vi "PH_Beckhoff_PP_PU.handle RRs.vi"(0 "i ref in":refnum<vi>, 4 "Values":T2, 5 "error in":errorcluster, 7 "Values changed at":T1) -> (14 "i ref out":refnum<vi>, 19 "error out":errorcluster)   [LabVIEW 2014, in "PH_Beckhoff_PP_PU.lvlib"]
doc: "This VI handles the incoming information about Ross Relais: The status is calculated and, if it changed, set to own attributes and published via DIM. All information is indicated at the GUI."
uses:
  PH_Beckhoff_PP_PU.lvlib
  PH_Beckhoff/PH_Beckhoff.Values.ctl
  PH_Beckhoff/PH_Beckhoff.Sonderklemmen Inputs.ctl
  PH_Beckhoff/PH_Beckhoff.Analog Inputs.ctl
  PH_Beckhoff/PH_Beckhoff.Scaling Type.ctl
  PH_Beckhoff/PH_Beckhoff.Analog Outputs.ctl
  PH_Beckhoff/PH_Beckhoff.Digital Inputs.ctl
  PH_Beckhoff/PH_Beckhoff.Digital Outputs.ctl
  PH_Basics/PH_StatusHandler/PH_StatusHandler.lvlib
  PH_Basics/PH_Common/PH_Common.lvlib
  PH_Beckhoff/PH_Beckhoff.lvlib
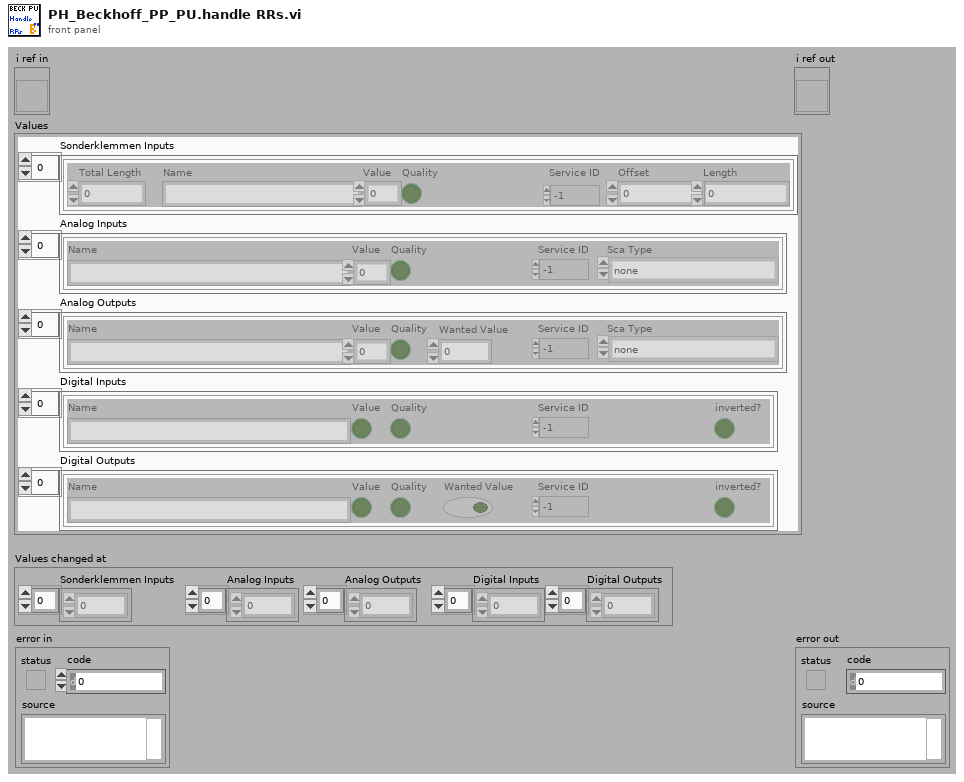
[diagram p1: front panel]
types:
  T1 = cluster{"Sonderklemmen Inputs":i32[], "Analog Inputs":i32[], "Analog Outputs":i32[], "Digital Inputs":i32[], "Digital Outputs":i32[]}
  T2 = typedef "PH_Beckhoff.lvlib/PH_Beckhoff.Values.ctl" = cluster{"Sonderklemmen Inputs":T3, "Analog Inputs":T4, "Analog Outputs":T6, "Digital Inputs":T7, "Digital Outputs":T8}
  T3 = typedef "PH_Beckhoff.lvlib/PH_Beckhoff.Sonderklemmen Inputs.ctl" = cluster{"Total Length":u32, "Name":string, "Value":u64, "Quality":bool, "Service ID":i32, "Offset":u32, "Length":u32}[]
  T4 = typedef "PH_Beckhoff.lvlib/PH_Beckhoff.Analog Inputs.ctl" = cluster{"Name":string, "Value":u32, "Quality":bool, "Service ID":i32, "Sca Type":T5}[]
  T5 = typedef "PH_Beckhoff.lvlib/PH_Beckhoff.Scaling Type.ctl" = enum16{"none", "0 ... 15 Bit -> 0 ... 5", "0 ... 15 Bit -> 0 ... 10", "0 ... 15 Bit -> 0 ... 25", "0 ... 15 Bit -> 4 ... 20", "0 ... 15 Bit -> 0 ... 1", "0 ... 15 Bit -> 0 ... 20000", "0 ... 15 Bit -> 0 ... 24000"}
  T6 = typedef "PH_Beckhoff.lvlib/PH_Beckhoff.Analog Outputs.ctl" = cluster{"Name":string, "Value":u32, "Quality":bool, "Wanted Value":u32, "Service ID":i32, "Sca Type":T5}[]
  T7 = typedef "PH_Beckhoff.lvlib/PH_Beckhoff.Digital Inputs.ctl" = cluster{"Name":string, "Value":bool, "Quality":bool, "Service ID":i32, "inverted?":bool}[]
  T8 = typedef "PH_Beckhoff.lvlib/PH_Beckhoff.Digital Outputs.ctl" = cluster{"Name":string, "Value":bool, "Quality":bool, "Wanted Value":bool, "Service ID":i32, "inverted?":bool}[]
  T9 = typedef "PH_Beckhoff_PP_PU.lvlib/PH_Beckhoff_PP_PU.i attribute.ctl" = cluster{"HV Meas":cluster{"Input GUI Ref":refnum<vi>, "Voltage Service ID":i32, "Voltage [V]":dbl, "Quality":bool, "# in Data":i32}[], "Trigger":cluster{"Status":cluster{"GUI Ref":refnum<vi>, "Status Service ID":i32, "Status":T10}, "last shot:":cluster{"GUI Ref":refnum<vi>, "Service ID":i32, "Time":string}, "DIs":cluster{"triggered":cluster{"GUI Ref":refnum<vi>, "# in Data":i32}, "fired":cluster{"GUI Ref":refnum<vi>, "# in Data":i32}}, "GUI Ref Indicator":refnum<vi>}[], "RR":cluster{"Status":cluster{"GUI Ref":refnum<vi>, "Status Service ID":i32, "Status":T10}, "DIs":cluster{"closed":cluster{"GUI Ref":refnum<vi>, "# in Data":i32}, "open":cluster{"GUI Ref":refnum<vi>, "# in Data":i32}}, "Close":cluster{"GUI Ref":refnum<vi>, "# in Data":i32}, "GUI Ref Indicator":refnum<vi>}[], "Igni":cluster{"Status":cluster{"GUI Ref":refnum<vi>, "Status Service ID":i32, "Status":T10}, "DIs":cluster{"heating on":cluster{"GUI Ref":refnum<vi>, "# in Data":i32}, "water on":cluster{"GUI Ref":refnum<vi>, "# in Data":i32}}, "Device on":cluster{"GUI Ref":refnum<vi>, "# in Data":i32}, "GUI Ref Indicator":refnum<vi>}[], "PSU":cluster{"Status":cluster{"GUI Ref":refnum<vi>, "Status Service ID":i32, "Status":T10}, "Limit Service ID":i32, "DIs":cluster{"inhibit":cluster{"GUI Ref":refnum<vi>, "# in Data":i32}, "end of charge":cluster{"GUI Ref":refnum<vi>, "# in Data":i32}, "HV on":cluster{"GUI Ref":refnum<vi>, "# in Data":i32}, "overtemp":cluster{"GUI Ref":refnum<vi>, "# in Data":i32}, "interlock":cluster{"GUI Ref":refnum<vi>, "# in Data":i32}, "load fault":cluster{"GUI Ref":refnum<vi>, "# in Data":i32}, "sum fault":cluster{"GUI Ref":refnum<vi>, "# in Data":i32}, "HV off":cluster{"GUI Ref":refnum<vi>, "# in Data":i32}, "DC ok":cluster{"GUI Ref":refnum<vi>, "# in Data":i32}}, "AIs":cluster{"voltage":cluster{"GUI Ref":refnum<vi>, "# in Data":i32}, "current":cluster{"GUI Ref":refnum<vi>, "# in Data":i32}}, "DAs":cluster{"inhibit":cluster{"GUI Ref":refnum<vi>, "# in Data":i32}, "interlock":cluster{"GUI Ref":refnum<vi>, "# in Data":i32}, "HV on":cluster{"GUI Ref":refnum<vi>, "# in Data":i32}, "Reset":cluster{"GUI Ref":refnum<vi>, "# in Data":i32}}, "AAs":cluster{"Voltage to set":cluster{"GUI Ref":refnum<vi>, "# in Data":i32}}, "GUI Ref Indicator":refnum<vi>}[], "reconfigured":cluster{"?":bool, "GUI Ref":refnum<vi>}, "PU Rack Type":T11, "HV Meas Info":T12, "PSU Info":T13}
  T10 = typedef "PH_StatusHandler.lvlib/PH_StatusHandler.Status.ctl" = i16
  T11 = typedef "PH_Beckhoff_PP_PU.lvlib/PH_Beckhoff_PP_PU.PU Rack Type.ctl" = enum16{"no Info", "PA 19mm", "PA 45mm", "MA PU 1 and 2", "MA PU 3 and 4", "MA PU 5 and 6", "MA FR and PILC"}
  T12 = typedef "PH_Beckhoff_PP_PU.lvlib/PH_Beckhoff_PP_PU.HV Meas Info.ctl" = cluster{"Period Time [s]":dbl, "Subtractor 1 [Hz]":dbl, "Devider 1 [Hz/kV]":dbl, "Subtractor 2 [Hz]":dbl, "Devider 2 [Hz/kV]":dbl}
  T13 = typedef "PH_Beckhoff_PP_PU.lvlib/PH_Beckhoff_PP_PU.PSU Info.ctl" = cluster{"Limits 1 [V]":cluster{"Lower":dbl, "Upper":dbl}, "Limits 2 [V]":cluster{"Lower":dbl, "Upper":dbl}}
  T14 = cluster{"Status":cluster{"GUI Ref":refnum<vi>, "Status Service ID":i32, "Status":T10}, "DIs":cluster{"closed":cluster{"GUI Ref":refnum<vi>, "# in Data":i32}, "open":cluster{"GUI Ref":refnum<vi>, "# in Data":i32}}, "Close":cluster{"GUI Ref":refnum<vi>, "# in Data":i32}, "GUI Ref Indicator":refnum<vi>}[]
  T15 = cluster{"Status":cluster{"GUI Ref":refnum<vi>, "Status Service ID":i32, "Status":T10}, "DIs":cluster{"closed":cluster{"GUI Ref":refnum<vi>, "# in Data":i32}, "open":cluster{"GUI Ref":refnum<vi>, "# in Data":i32}}, "Close":cluster{"GUI Ref":refnum<vi>, "# in Data":i32}, "GUI Ref Indicator":refnum<vi>}
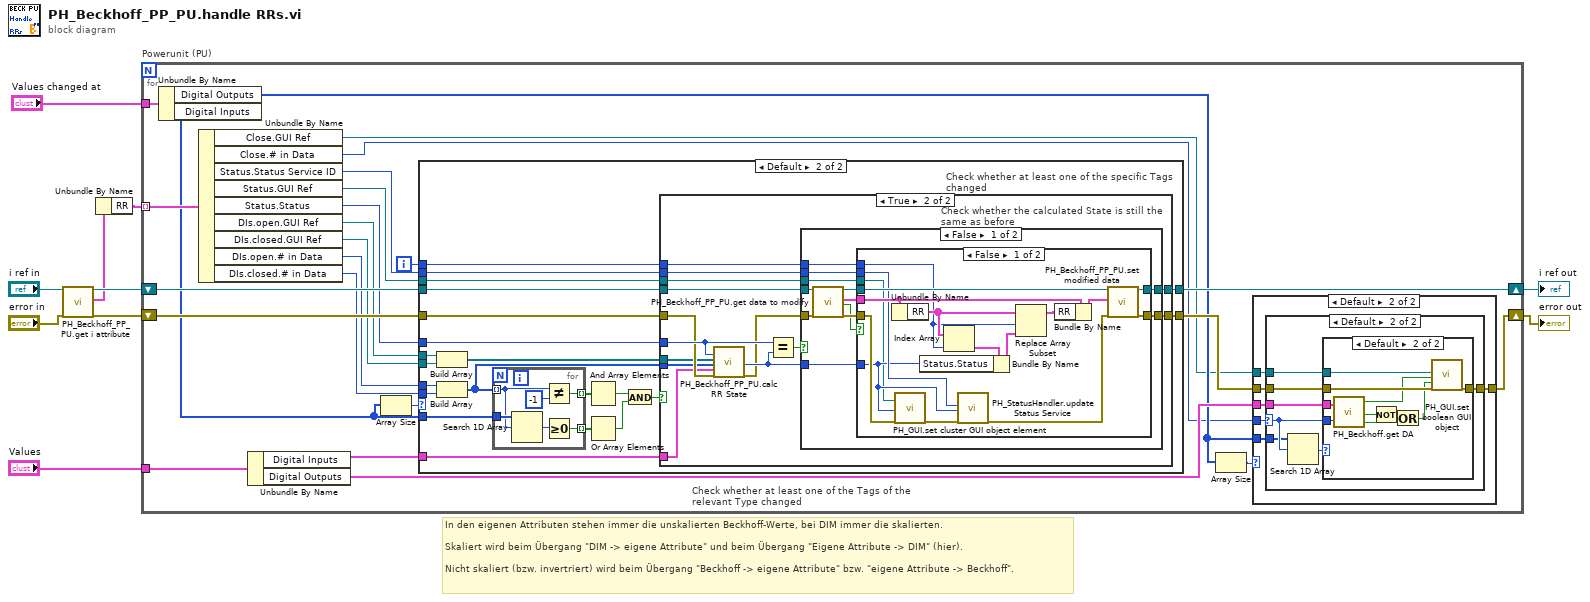
[diagram p0: block diagram]
diagram:
  # "In den eigenen Attributen stehen immer die unskalierten Beckhoff-Werte, bei DIM immer die skalierten.\n\nSkaliert wird beim Übergang \"DIM -> eigene Attribute\" und beim Übergang \"Eigene Attribute -> DIM\" (hier).\n\nNicht skaliert (bzw. invertriert) wird beim Übergang \"Beckhoff -> eigene Attribute\" bzw. \"eigene Attribute -> Beckhoff\"."
  n1 = call "PH_Beckhoff_PP_PU.get i attribute.vi"("i ref in"="i ref in", "error in (no error)"="error in") -> ("i ref out"=w6:refnum<vi>, "i attribute"=w4:T9, "error out"=w5:errorcluster)  [unwired: 15 in]
  n2 = Unbundle By Name(w4) -> ("RR"=w3:T14)
  n3 = for "Powerunit (PU)" {
    shift-right: [w18] -> w7
    shift-left: w5 -> [w29]
    tunnel: w3 -> [w34] mode=indexing
    shift-right: [w30] -> w8
    shift-left: w6 -> [w32]
    tunnel: "Values" -> [w21]
    tunnel: "Values changed at" -> [w23]
    i -> [w31]
    n4 = Unbundle By Name(w23) -> ("Digital Outputs"=w15:i32[], "Digital Inputs"=w20:i32[])
    n5 = Unbundle By Name(w34) -> ("Close.GUI Ref"=w11:refnum<vi>, "Close.# in Data"=w14:i32, "Status.Status Service ID"=w33:i32, "Status.GUI Ref"=w25:refnum<vi>, "Status.Status"=w28:T10, "DIs.open.GUI Ref"=w27:refnum<vi>, "DIs.closed.GUI Ref"=w26:refnum<vi>, "DIs.open.# in Data"=w13:i32, "DIs.closed.# in Data"=w12:i32)
    n6 = Unbundle By Name(w21) -> ("Digital Inputs"=w22:T7, "Digital Outputs"=w17:T8)
    n7 = Array Size(array=w20) -> (size(s)=w24:i32)
    n8 = case "Check whether at least one of the Tags of the relevant Type changed" shown="Default" w24 {
      tunnel: w33 -> [_ w83]
      tunnel: w32 -> [w62 w82]
      tunnel: w31 -> [_ w81]
      tunnel: [w62 w80] -> w30
      tunnel: [w61 w79] -> w19
      tunnel: w22 -> [_ w78]
      tunnel: w29 -> [w61 w77]
      tunnel: w13 -> [_ w76]
      tunnel: w12 -> [_ w75]
      tunnel: w20 -> [_ w73]
      tunnel: w28 -> [_ w67]
      tunnel: w27 -> [_ w66]
      tunnel: w26 -> [_ w65]
      tunnel: w25 -> [_ w63]
      frame 0 {
      }
      frame Default {
        n9 = Build Array(w66, w65) -> (w64:refnum<vi>[])
        n10 = Build Array(w76, w75) -> (w74:i32[])
        n11 = for {
          tunnel: w74 -> [w135] mode=indexing
          tunnel: [w137] -> w72 mode=indexing
          tunnel: w73 -> [w136]
          tunnel: [w132] -> w70 mode=indexing
          n12 = Search 1D Array(1D array=w136, element=w135) -> (index of element=w133:i32)  [unwired: 1 in]
          n13 = Not Equal?(x=w135, y=-1) -> (x != y?=w137:bool)
          n14 = Greater Or Equal To 0?(x=w133) -> (x >= 0?=w132:bool)
        }
        n15 = And Array Elements(Boolean array=w72) -> (logical AND=w71:bool)
        n16 = Or Array Elements(Boolean array=w70) -> (logical OR=w69:bool)
        n17 = And(x=w71, y=w69) -> (x .and. y?=w68:bool)
        n18 = case "Check whether at least one of the specific Tags changed" shown="True" w68 {
          tunnel: w83 -> [_ w99]
          tunnel: w82 -> [w85 w98]
          tunnel: w81 -> [_ w97]
          tunnel: [w85 w95] -> w80
          tunnel: [w84 w94] -> w79
          tunnel: w78 -> [_ w88]
          tunnel: w67 -> [_ w92]
          tunnel: w77 -> [w84 w89]
          tunnel: w74 -> [_ w87]
          tunnel: w64 -> [_ w86]
          tunnel: w63 -> [_ w93]
          frame False {
          }
          frame True {
            n19 = call "PH_Beckhoff_PP_PU.calc RR State.vi"("old RR Status"=w92, "GUI Refs: open and closed"=w86, "# in Data: open and closed"=w87, "Digital Inputs"=w88, "error in"=w89) -> ("Ross Relais Status"=w91:T10, "error out"=w90:errorcluster)  [unwired: 13 in]
            n20 = Equal?(x=w92, y=w91) -> (x = y?=w96:bool)
            n21 = case "Check whether the calculated State is still the same as before" shown="False" w96 {
              tunnel: [w106 w130] -> w94
              tunnel: w99 -> [w111 _]
              tunnel: w90 -> [w110 w130]
              tunnel: w91 -> [w109 _]
              tunnel: w98 -> [w107 w131]
              tunnel: [w104 w131] -> w95
              tunnel: w97 -> [w102 _]
              tunnel: w93 -> [w100 _]
              frame False {
                n22 = call "PH_Beckhoff_PP_PU.get data to modify.vi"("i ref in"=w107, "error in (no error)"=w110) -> ("i ref out"=w105:refnum<vi>, "i attribute"=w103:T9, "timed out"=w101:bool, "error out"=w108:errorcluster)  [unwired: 14 in]
                n23 = case shown="False" w101 {
                  tunnel: w111 -> [w116 _]
                  tunnel: w109 -> [w113 _]
                  tunnel: w108 -> [w115 w128]
                  tunnel: [w127 w128] -> w106
                  tunnel: w105 -> [w126 w129]
                  tunnel: [w125 w129] -> w104
                  tunnel: w103 -> [w124 _]
                  tunnel: w102 -> [w120 _]
                  tunnel: w100 -> [w112 _]
                  frame False {
                    n24 = Unbundle By Name(w124) -> ("RR"=w121:T14)
                    n25 = call "PH_GUI.set cluster GUI object element.vi"("Ctl Refnum"=w112, "Value"=w113, "error in"=w115) -> ("error out"=w114:errorcluster)  [unwired: 16 in]
                    n26 = Index Array(array=w121, index=w120) -> (element=w119:T15)
                    n27 = Bundle By Name(cluster=w119, "Status.Status"=w113) -> (w118:T15)
                    n28 = call "PH_StatusHandler.update Status Service.vi"("Service ID"=w116, "Status"=w113, "error in (no error)"=w114) -> ("error out"=w117:errorcluster)  [unwired: 16 in]
                    n29 = Replace Array Subset(array=w121, new element=w118, index=w120) -> (w122:T14)
                    n30 = Bundle By Name(cluster=w124, "RR"=w122) -> (w123:T9)
                    n31 = call "PH_Beckhoff_PP_PU.set modified data.vi"("i ref in"=w126, "i attribute"=w123, "error in (no error)"=w117) -> ("i ref out"=w125:refnum<vi>, "error out"=w127:errorcluster)  [unwired: 15 in]
                  }
                  frame True {
                  }
                }
              }
              frame True {
              }
            }
          }
        }
      }
    }
    n32 = Array Size(array=w15) -> (size(s)=w16:i32)
    n33 = case shown="Default" w16 {
      tunnel: w19 -> [w35 w41]
      tunnel: [w35 w40] -> w18
      tunnel: w17 -> [_ w39]
      tunnel: w11 -> [_ w38]
      tunnel: w14 -> [_ w37]
      tunnel: w15 -> [_ w36]
      frame 0 {
      }
      frame Default {
        n34 = case shown="Default" w37 {
          selector: w37 -> [_ w45]
          tunnel: w41 -> [w42 w49]
          tunnel: [w42 w48] -> w40
          tunnel: w39 -> [_ w47]
          tunnel: w38 -> [_ w46]
          tunnel: w36 -> [_ w44]
          frame -1 {
          }
          frame Default {
            n35 = Search 1D Array(1D array=w44, element=w45) -> (index of element=w43:i32)  [unwired: 1 in]
            n36 = case shown="Default" w43 {
              tunnel: w49 -> [w50 w60]
              tunnel: [w50 w59] -> w48
              tunnel: w47 -> [_ w58]
              tunnel: w46 -> [_ w57]
              tunnel: w45 -> [_ w51]
              frame -1 {
              }
              frame Default {
                n37 = call "PH_Beckhoff.get DA.vi"("Digital Outputs"=w58, "index of element"=w51) -> ("Value"=w56:bool, "Quality"=w53:bool, "Tag not found"=w54:bool)
                n38 = Not(x=w53) -> (.not. x?=w52:bool)
                n39 = Or(x=w52, y=w54) -> (x .or. y?=w55:bool)
                n40 = call "PH_GUI.set boolean GUI object.vi"("Boolean Knob GUI Ref"=w57, "Value"=w56, "Blinking? (false)"=w55, "error in (no error)"=w60) -> ("error out"=w59:errorcluster)  [unwired: 15 in]
              }
            }
          }
        }
      }
    }
  }
  "error out" <- w7
  "i ref out" <- w8
